vi "oa_Extract Even Angle Signal by Indice(1 CH).vi"(0 "even angle signal":cluster{"r0":dbl, "dr":dbl, "Y":dbl[]}={"r0"=0.0, "dr"=1.0, "Y"=[]} {"r0" format="%.2p"; "dr" format="%.2p"; "Y" format="%.2f"}, 1 "reset?":bool, 7 "trigger indices":T1, 11 "block size":i32=1024 min=2, 12 "indices end?":bool) -> (3 "new signal available?":bool, 4 "even angle signal output":cluster{"r0":dbl, "dr":dbl, "Y":dbl[]}, 14 "reached end?":bool, 15 "current positon":cluster{"rev":dbl, "time":dbl, "RPM":dbl})   [LabVIEW 2017, in "SoundVib_OAUtility.lvlib"]
uses:
  <vilib>/addons/Sound and Vibration/Order Analysis/Utility/SoundVib_OAUtility.lvlib
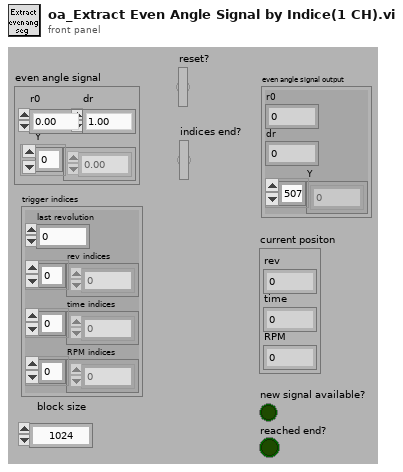
[diagram p1: front panel]
types:
  T1 = cluster{"last revolution":dbl, "rev indices":dbl[], "time indices":dbl[], "RPM indices":dbl[]}
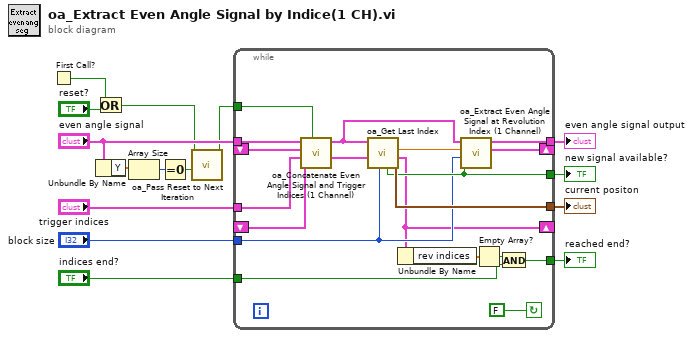
[diagram p0: block diagram]
diagram:
  n1 = First Call?() -> (First Call?: T/F=w9:bool)
  n2 = Or(x=w9, y="reset?") -> (x .or. y?=w7:bool)
  n3 = Unbundle By Name("even angle signal") -> ("Y"=w13:dbl[])
  n4 = Array Size(array=w13) -> (size(s)=w12:i32)
  n5 = Equal To 0?(x=w12) -> (x = 0?=w10:bool)
  n6 = call <vilib>:"oa_Pass Reset to Next Iteration.vi"("trigger"=w10, "reset?(F)"=w7) -> ("reset out"=w6:bool)  [unwired: 9 in]
  n7 = while {
    tunnel: w6 -> [w29]
    shift-right: [w23] -> _
    shift-left: _ -> [w31]
    tunnel: "even angle signal" -> [w30]
    tunnel: "block size" -> [w21]
    tunnel: "trigger indices" -> [w32]
    shift-right: [w20] -> _
    shift-left: _ -> [w33]
    tunnel: [w27] -> w5
    tunnel: [w24] -> w4
    tunnel: [w22] -> w3
    tunnel: "indices end?" -> [w17]
    tunnel: [w16] -> w1
    stop <- FALSE continue-if-true
    n8 = call <vilib>:"oa_Concatenate Even Angle Signal and Trigger Indices (1 Channel).vi"("reset?"=w29, "history trigger indices"=w33, "trigger indices"=w32, "history even angle signal"=w31, "even angle signal"=w30) -> ("trigger indices out"=w28:T1, "even angle signal out"=w26:cluster{"r0":dbl, "dr":dbl, "Y":dbl[]})  [unwired: 5 in]
    n9 = call <vilib>:"oa_Get Last Index.vi"("block size"=w21, "trigger indices"=w28, "even angle signal"=w26) -> ("current positon"=w27:cluster{"rev":dbl, "time":dbl, "RPM":dbl}, "trigger indices for buffer"=w20:T1, "rev index"=w25:dbl, "index in range"=w22:bool)  [unwired: 5 in]
    n10 = Unbundle By Name(w20) -> ("rev indices"=w19:dbl[])
    n11 = call <vilib>:"oa_Extract Even Angle Signal at Revolution Index (1 Channel).vi"("index in range"=w22, "block size"=w21, "rev index"=w25, "even angle signal"=w26) -> ("even angle signal for buffer"=w23:cluster{"r0":dbl, "dr":dbl, "Y":dbl[]}, "even angle signal out"=w24:cluster{"r0":dbl, "dr":dbl, "Y":dbl[]})  [unwired: 6 in]
    n12 = Empty Array?(array=w19) -> (empty?=w18:bool)
    n13 = And(x=w18, y=w17) -> (x .and. y?=w16:bool)
  }
  "even angle signal output" <- w4
  "current positon" <- w5
  "new signal available?" <- w3
  "reached end?" <- w1
